vi "Project Item Recursion.vi"(8 "error in":errorcluster, 11 "TargetItem in":refnum<vi>) -> (0 "error out":errorcluster, 3 "TargetItem out":refnum<vi>[](array[refnum]))   [LabVIEW 2023, in "Plugin Generator.lvlib"]
uses:
  Plugin Generator.lvlib
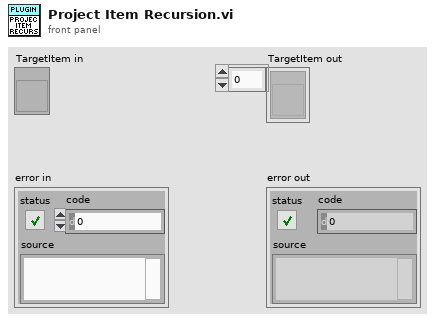
[diagram p1: front panel]
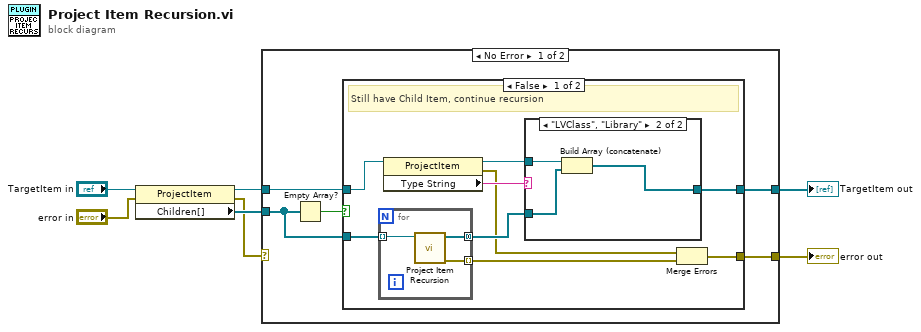
[diagram p0: block diagram]
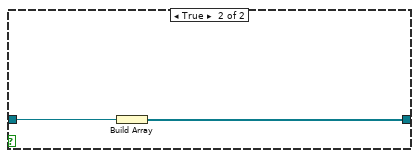
[diagram p3: hidden frame]
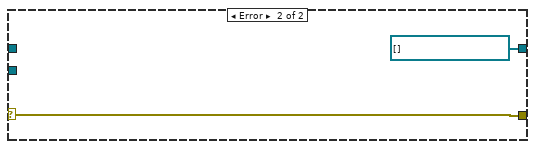
[diagram p4: hidden frame]
diagram:
  n1 = property class="ProjectItem"(reference="TargetItem in", error in="error in") -> (reference out=w3:refnum<vi>, error out=w1:errorcluster, "Children[]"=w2:refnum<vi>[])
  n2 = case shown="No Error" w1 {
    selector: w1 -> [_ w31]
    tunnel: [w12 refnum<vi>[] [] ("TargetItem out")] -> w7
    tunnel: [w11 w31] -> w5
    tunnel: w3 -> [w9 _]
    tunnel: w2 -> [w8 _]
    frame No Error {
      n3 = Empty Array?(array=w8) -> (empty?=w10:bool)
      n4 = case shown="False" w10 {
        tunnel: [w14 w29] -> w12
        tunnel: w9 -> [w18 w30]
        tunnel: w8 -> [w21 _]
        tunnel: [w19 _] -> w11
        frame False {
          # "Still have Child Item, continue recursion"
          n5 = for {
            tunnel: w21 -> [w27] mode=indexing
            tunnel: [w28] -> w16 mode=concatenating
            tunnel: [w26] -> w20 mode=indexing
            n6 = call "Project Item Recursion.vi"("TargetItem in"=w27) -> ("error out"=w26:errorcluster, "TargetItem out"=w28:refnum<vi>[])  [unwired: 9 in]
          }
          n7 = property class="ProjectItem"(reference=w18) -> (reference out=w15:refnum<vi>, error out=w13:errorcluster, "Type String"=w17:string)  [unwired: 1 in]
          n8 = case shown="\"LVClass\", \"Library\"" w17 {
            tunnel: w16 -> [w22 w25]
            tunnel: w15 -> [_ w24]
            tunnel: [w22 w23] -> w14
            frame Default {
              # "Not target type of item"
            }
            frame "LVClass", "Library" {
              n9 = Build Array (concatenate)(w24, w25) -> (w23:refnum<vi>[])
            }
          }
          n10 = Merge Errors(w13, w20) -> (w19:errorcluster)
        }
        frame True {
          n11 = Build Array(w30) -> (w29:refnum<vi>[])
        }
      }
    }
    frame Error {
    }
  }
  "TargetItem out" <- w7
  "error out" <- w5
